vi "Main VIm.vi"() -> ()   [LabVIEW 2012]
panel:
  in  "Run next SubVI":bool
  in  "Sent Polarizer":bool
  in  "stop":bool
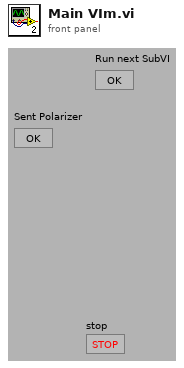
[diagram p1: front panel]
types:
  T1 = cluster{"Counter Pol":i32, "Analyser":dbl, "X":dbl[], "Y":dbl[]}
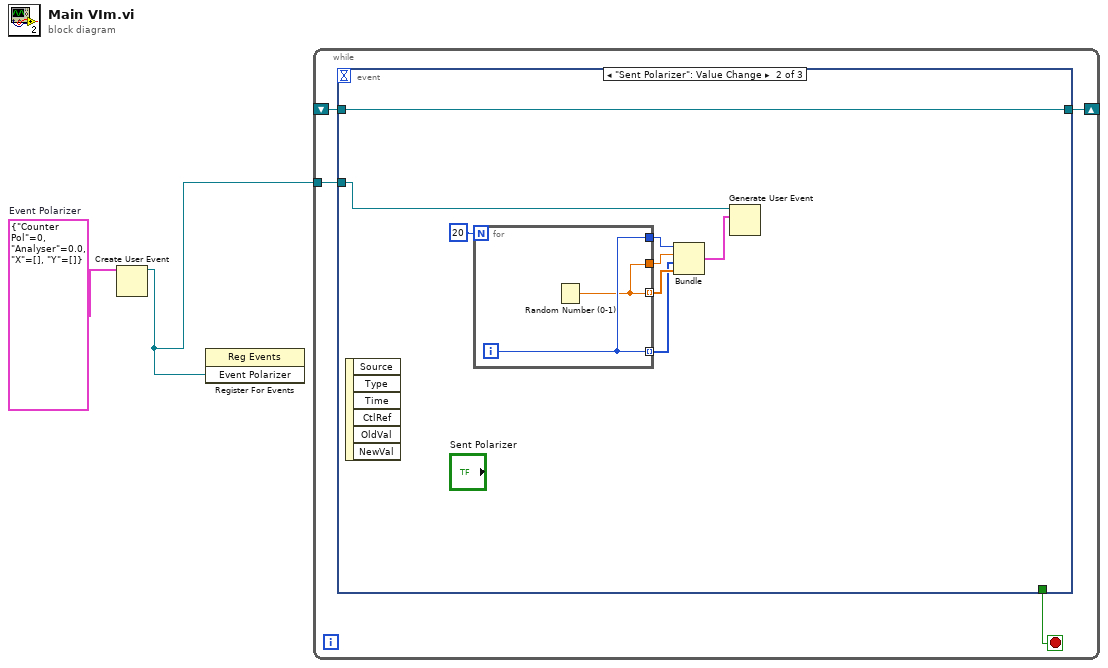
[diagram p0: block diagram]
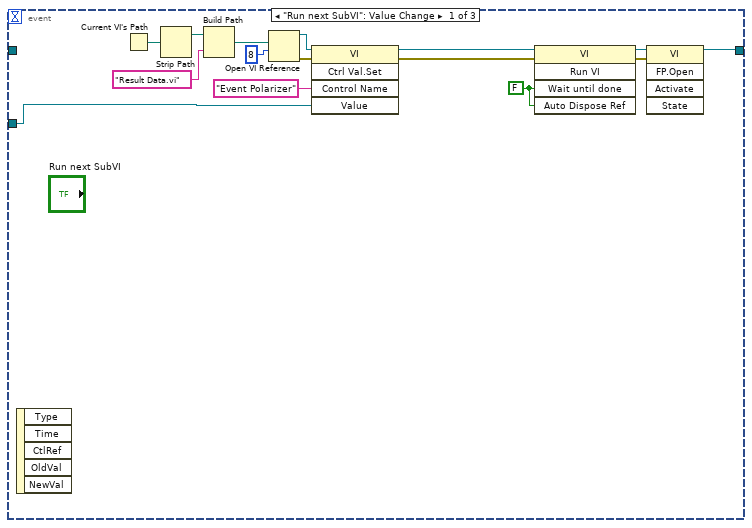
[diagram p2: hidden frame]
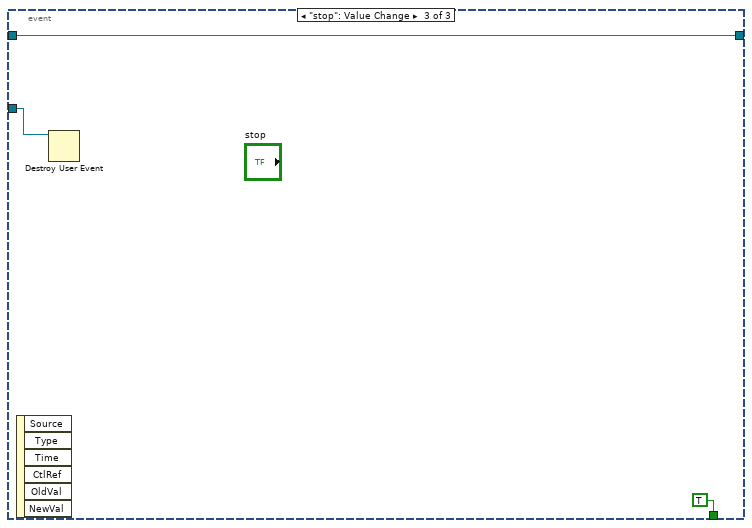
[diagram p3: hidden frame]
diagram:
  w2 = T1 {"Counter Pol"=0, "Analyser"=0.0, "X"=[], "Y"=[]}  # Event Polarizer
  n1 = Create User Event(user event datatype=w2) -> (user event=w1:refnum<user-event>)  [unwired: 1 in, 1 out]
  n2 = register-events(w1) -> ()  [unwired: 2 in, 2 out]
  n3 = while {
    tunnel: w1 -> [w6]
    shift-right: [w4] -> _
    shift-left: _ -> [w3]
    stop <- w5 stop-if-true
    n4 = event shown="[1] \"Sent Polarizer\": Value Change" {
      selector: _ -> [_ _ _]
      dyn-events: _ -> [_ _ _]
      timeout: _ -> [_ _ _]
      tunnel: w6 -> [w10 w24 w32]
      tunnel: [_ _ TRUE] -> w5
      tunnel: [w9 w22 w33] -> w4
      tunnel: w3 -> [_ w22 w33]
      event "Run next SubVI": Value Change {
        w19 = FALSE ("Wait Until Done")
        n5 = event-data() -> ()  [unwired: 6 out]
        n6 = Current VI's Path() -> (path=w11:path)
        n7 = Strip Path(path=w11) -> (stripped path=w12:path)  [unwired: 1 out]
        n8 = Build Path(base path=w12, name or relative path="Result Data.vi") -> (appended path=w14:path)
        n9 = Open VI Reference(vi path=w14, options=8) -> (vi reference=w16:refnum<vi>, error out=w17:errorcluster)  [unwired: 1 in, 3 out]
        n10 = invoke class="VI" method="Ctrl Val.Set"(reference=w16, error in=w17, "Control Name"="Event Polarizer", "Value"=w10) -> (reference out=w8:refnum<vi>, error out=w7:errorcluster)  [unwired: 1 in, 3 out]
        n11 = invoke class="VI" method="Run VI"(reference=w8, error in=w7, "Wait until done"=w19, "Auto Dispose Ref"=w19) -> (reference out=w21:refnum<vi>, error out=w20:errorcluster)  [unwired: 1 in, 3 out]
        n12 = invoke class="VI" method="FP.Open"(reference=w21, error in=w20) -> (reference out=w9:refnum<vi>)  [unwired: 3 in, 4 out]
      }
      event "Sent Polarizer": Value Change {
        n13 = event-data() -> ()  [unwired: 7 out]
        n14 = for {
          N: 20 -> [_]
          tunnel: [w30] -> w26 mode=indexing
          tunnel: [w31] -> w25 mode=indexing
          tunnel: [w31] -> w28
          tunnel: [w30] -> w27
          i -> [w31]
          n15 = Random Number (0-1)() -> (number: 0 to 1=w30:dbl)
        }
        n16 = Bundle(w28, "number: 0 to 1"=w27, w25, w26) -> (w23:cluster{i32, "number: 0 to 1":dbl, i32[], dbl[]})  [unwired: 1 out]
        n17 = Generate User Event(user event=w24, event data cluster=w23) -> ()  [unwired: 1 in, 2 out]
      }
      event "stop": Value Change {
        n18 = event-data() -> ()  [unwired: 7 out]
        n19 = Destroy User Event(user event=w32) -> ()  [unwired: 1 in, 1 out]
      }
    }
  }
